vi "RP Write Command TCP.vi"(6 "timeout ms (25000)":i32=1000, 7 "Config offset":u64, 8 "Error In":errorcluster, 9 "Command payload":u64 format="%x", 10 "Command number":T1, 11 "connection ID":refnum<k5>) -> (0 "Error Out":errorcluster, 2 "bytes written":i32, 3 "connection ID out":refnum<k5>)   [LabVIEW 2019]
uses:
  RP Command.ctl
panel:
  out "x .or. y?":u64 format="%x"
  out "x << y":u64 format="%x"
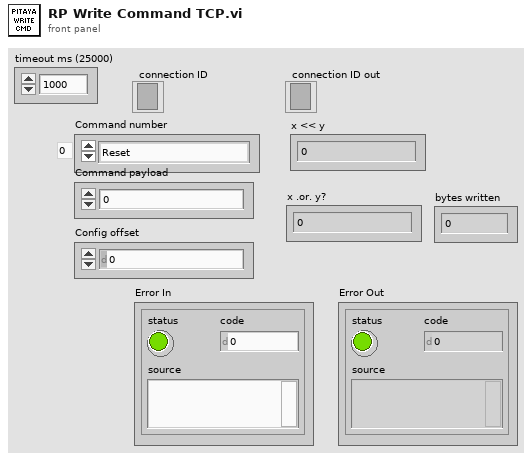
[diagram p1: front panel]
types:
  T1 = typedef "RP Command.ctl" = enum16{"Reset", "Read IDN", "Stop server", "Get status", "Get temperature", "Connect client", "Arm", "Software trigger", "Get whole buffer", "Get chunk", "System call", "Get config", "Set config", "Recieve data", "Recieve Calibartion", "Transmit data"}
  T2 = enum16{"big-endian, network order", "native, host order", "little-endian"}
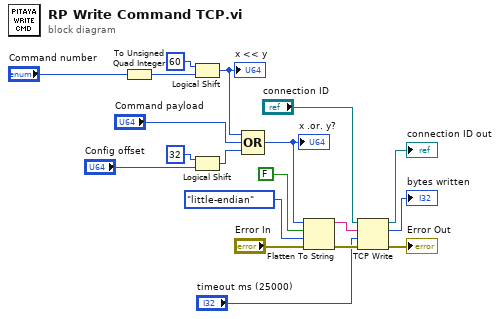
[diagram p0: block diagram]
diagram:
  n1 = To Unsigned Quad Integer(1:"Command number") -> (0:w5:u64)
  n2 = Logical Shift(y=i16 60, x=w5) -> (x << y=w17:u64)
  "x << y" <- w17
  n3 = Logical Shift(y=i16 32, x="Config offset") -> (x << y=w2:u64)
  n4 = Compound Arithmetic op=OR(w17, "Command payload", w2) -> (w7:u64)
  "x .or. y?" <- w7
  n5 = Flatten To String(anything=w7, prepend array or string size? (T)=FALSE, byte order (0:big-endian, network order)=T2."little-endian", error in (no error)="Error In") -> (data string=w11:string, error out=w12:errorcluster)  [unwired: 1 out]
  n6 = TCP Write(connection ID="connection ID", data in=w11, error in (no error)=w12, 9:"timeout ms (25000)") -> (connection ID out=→"connection ID out":refnum<k5>, bytes written=→"bytes written":i32, error out=→"Error Out":errorcluster)
